vi "Ex4 Grayscalling.vi"() -> ()   [LabVIEW 2020]
panel:
  in  "Final Image Type":T1 items=["Grayscale (U8)", "Grayscale (I16)", "Grayscale (SGL)", "Complex (CSG)", "RGB (U32)", "HSL (U32)", "RGB (U64)", "Grayscale (U16)"]
  out "error out":errorcluster
  in  "Color Channel 2":string(combo)
  out "Color Channel":T2(plugin-control)
  out "Image":T2(plugin-control)
  in  "Source Image Type":T1 items=["Grayscale (U8)", "Grayscale (I16)", "Grayscale (SGL)", "Complex (CSG)", "RGB (U32)", "HSL (U32)", "RGB (U64)", "Grayscale (U16)"]
  in  "File Path":path
  # "EX.4 GRAYSCALLING"
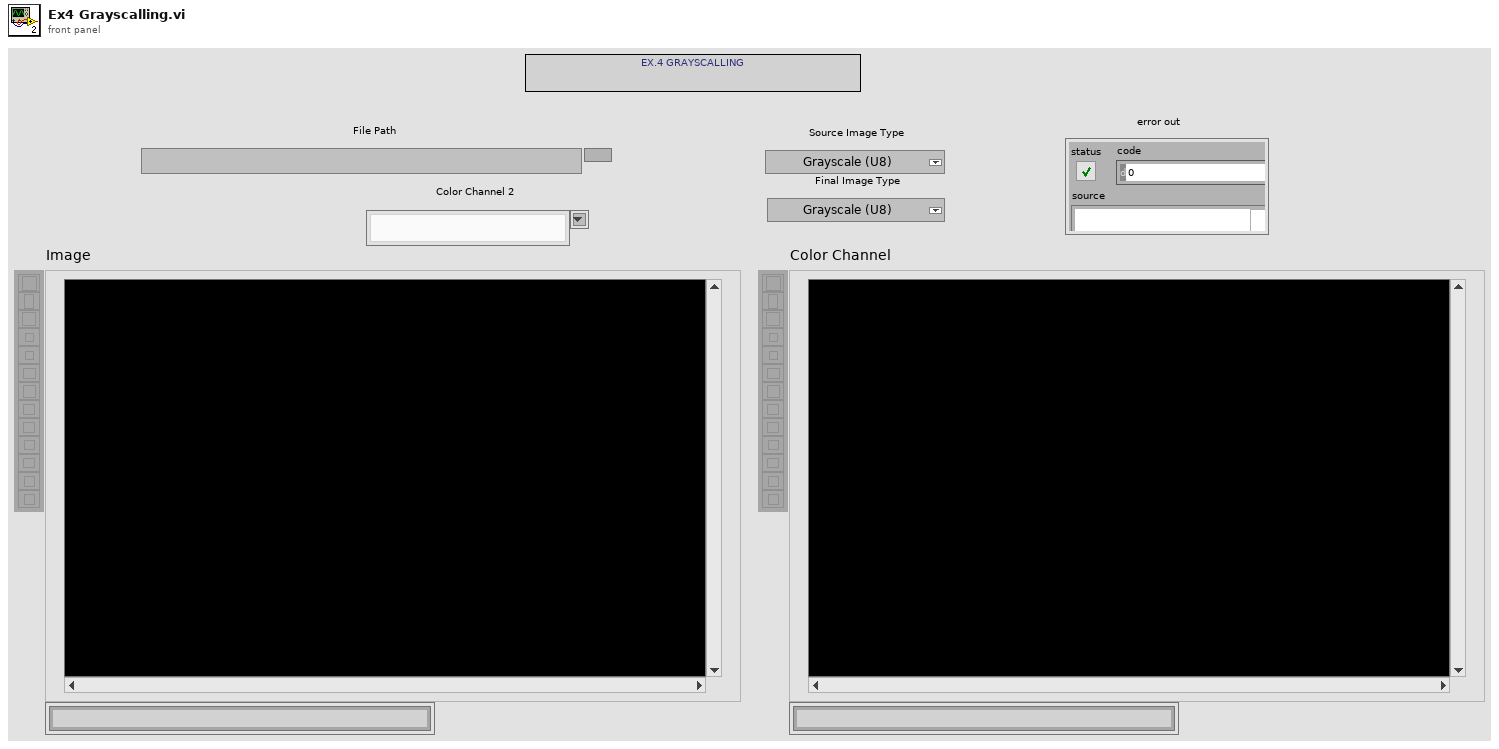
[diagram p1: front panel]
types:
  T1 = typedef "Image Type" = u32
  T2 = typedef "IMAQ Image.ctl" = refnum<image>
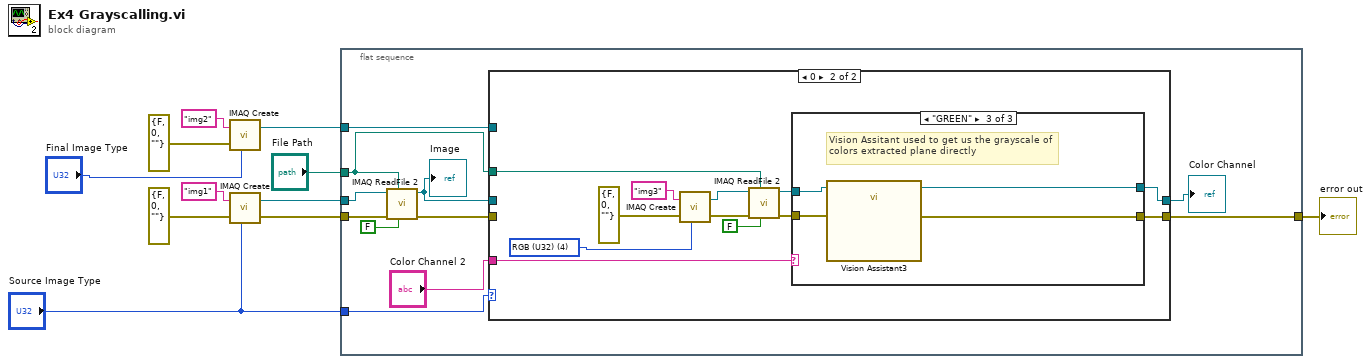
[diagram p0: block diagram]
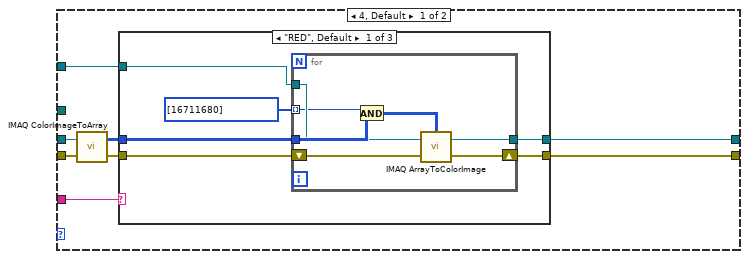
[diagram p2: hidden frame]
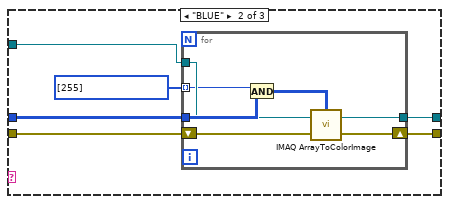
[diagram p3: hidden frame]
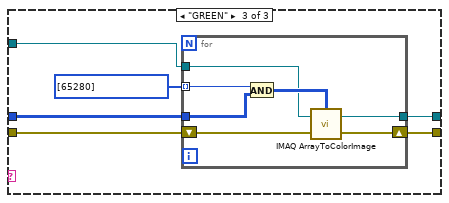
[diagram p4: hidden frame]
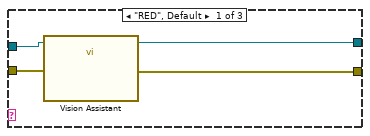
[diagram p5: hidden frame]
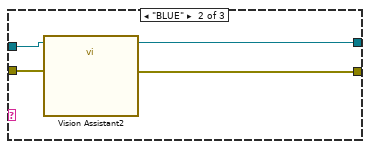
[diagram p6: hidden frame]
diagram:
  n1 = call "IMAQ Create"("Image Name"="img2", "Image Type"="Final Image Type", "error in (no error)"=errorcluster {"status"=FALSE, "code"=0, "source"=""}) -> ("New Image"=w5:T2)  [unwired: 2 in, 1 out]
  n2 = call "IMAQ Create"("Image Name"="img1", "Image Type"="Source Image Type", "error in (no error)"=errorcluster {"status"=FALSE, "code"=0, "source"=""}) -> ("New Image"=w2:T2, "error out"=w3:errorcluster)  [unwired: 2 in]
  n3 = flat-sequence {
    tunnel: "Source Image Type" -> [w18]
    tunnel: w5 -> [w17]
    tunnel: "File Path" -> [w15]
    tunnel: w3 -> [w14]
    tunnel: w2 -> [w13]
    tunnel: [w12] -> w1
    frame #0 {
      n4 = call "IMAQ ReadFile 2"("Use File Path Image Type"=FALSE, "File Path"=w15, "error in (no error)"=w14, "Image"=w13) -> ("error out"=w22:errorcluster, "Image Out"=w21:T2)  [unwired: 3 in, 3 out]
      "Image" <- w21
      n5 = case shown="0" w18 {
        tunnel: w17 -> [w28 _]
        tunnel: [w27 w79] -> w19
        tunnel: [w26 w80] -> w12
        tunnel: "Color Channel 2" -> [w25 w81]
        tunnel: w15 -> [_ w72]
        tunnel: w21 -> [w24 _]
        tunnel: w22 -> [w23 _]
        frame 4, Default {
          n6 = call "IMAQ ColorImageToArray"("Image"=w24, "error in (no error)"=w23) -> ("Image Pixels (U32)"=w29:u32[][], "error out"=w30:errorcluster)  [unwired: 2 in, 1 out]
          n7 = case shown="\"RED\", Default" w25 {
            tunnel: w29 -> [w35 w46 w62]
            tunnel: w30 -> [w33 w48 w61]
            tunnel: w28 -> [w34 w47 w60]
            tunnel: [w32 w45 w58] -> w27
            tunnel: [w31 w44 w57] -> w26
            frame "RED", Default {
              n8 = for {
                tunnel: w35 -> [w43]
                shift-right: [w40] -> w31
                shift-left: w33 -> [w41]
                tunnel: [w39] -> w32
                tunnel: w34 -> [w38]
                tunnel: i32[] [16711680] -> [w37] mode=indexing
                n9 = And(x=w37, y=w43) -> (x .and. y?=w42:u32[][])
                n10 = call "IMAQ ArrayToColorImage"("Image Pixels (U32)"=w42, "Image"=w38, "error in (no error)"=w41) -> ("Image Out"=w39:T2, "error out"=w40:errorcluster)  [unwired: 2 in]
              }
            }
            frame "BLUE" {
              n11 = for {
                tunnel: w46 -> [w56]
                shift-right: [w53] -> w44
                shift-left: w48 -> [w54]
                tunnel: [w52] -> w45
                tunnel: w47 -> [w51]
                tunnel: i32[] [255] -> [w50] mode=indexing
                n12 = And(x=w50, y=w56) -> (x .and. y?=w55:u32[][])
                n13 = call "IMAQ ArrayToColorImage"("Image Pixels (U32)"=w55, "Image"=w51, "error in (no error)"=w54) -> ("Image Out"=w52:T2, "error out"=w53:errorcluster)  [unwired: 2 in]
              }
            }
            frame "GREEN" {
              n14 = for {
                tunnel: w62 -> [w69]
                shift-right: [w66] -> w57
                shift-left: w61 -> [w67]
                tunnel: [w65] -> w58
                tunnel: w60 -> [w64]
                tunnel: i32[] [65280] -> [w63] mode=indexing
                n15 = And(x=w63, y=w69) -> (x .and. y?=w68:u32[][])
                n16 = call "IMAQ ArrayToColorImage"("Image Pixels (U32)"=w68, "Image"=w64, "error in (no error)"=w67) -> ("Image Out"=w65:T2, "error out"=w66:errorcluster)  [unwired: 2 in]
              }
            }
          }
        }
        frame 0 {
          w76 = T1 4 items=["Grayscale (U8)", "Grayscale (I16)", "Grayscale (SGL)", "Complex (CSG)", "RGB (U32)", "HSL (U32)", "RGB (U64)", "Grayscale (U16)"] ("Image Type")
          n17 = call "IMAQ Create"("Image Name"="img3", "Image Type"=w76, "error in (no error)"=errorcluster {"status"=FALSE, "code"=0, "source"=""}) -> ("New Image"=w75:T2, "error out"=w74:errorcluster)  [unwired: 2 in]
          n18 = call "IMAQ ReadFile 2"("Use File Path Image Type"=FALSE, "File Path"=w72, "error in (no error)"=w74, "Image"=w75) -> ("error out"=w70:errorcluster, "Image Out"=w71:T2)  [unwired: 3 in, 3 out]
          n19 = case shown="\"GREEN\"" w81 {
            tunnel: w71 -> [w85 w89 w90]
            tunnel: w70 -> [w84 w87 w93]
            tunnel: [w83 w86 w91] -> w80
            tunnel: [w82 w88 w92] -> w79
            frame "RED", Default {
              n20 = call "Vision Assistant"("Image In"=w85, "error in"=w84) -> ("Image Out"=w82:T2, "error out"=w83:errorcluster)  [unwired: 24 in]
            }
            frame "BLUE" {
              n21 = call "Vision Assistant2"("Image In"=w89, "error in"=w87) -> ("Image Out"=w88:T2, "error out"=w86:errorcluster)  [unwired: 24 in]
            }
            frame "GREEN" {
              # "Vision Assitant used to get us the grayscale of colors extracted plane directly"
              n22 = call "Vision Assistant3"("Image In"=w90, "error in"=w93) -> ("Image Out"=w92:T2, "error out"=w91:errorcluster)  [unwired: 24 in]
            }
          }
        }
      }
      "Color Channel" <- w19
    }
  }
  "error out" <- w1
